vi "5790A acdc unit.vi"(6 "error in":errorcluster, 8 "unit":enum16{"ppm", "pct", "V", "ratio"}(ring), 9 "5790A":refnum<visa-resource-name>) -> (0 "error out":errorcluster, 3 "Session Out":refnum<visa-resource-name>)   [LabVIEW 2009]
uses:
  <vilib>/Instr/_visa.llb/VISA GPIB Control REN Mode.ctl
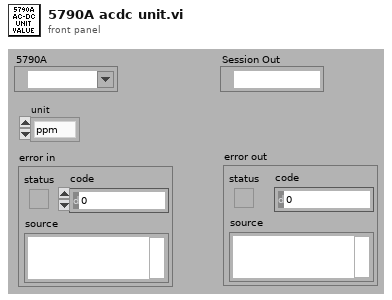
[diagram p1: front panel]
types:
  T1 = typedef "VISA GPIB Control REN Mode.ctl" = u16
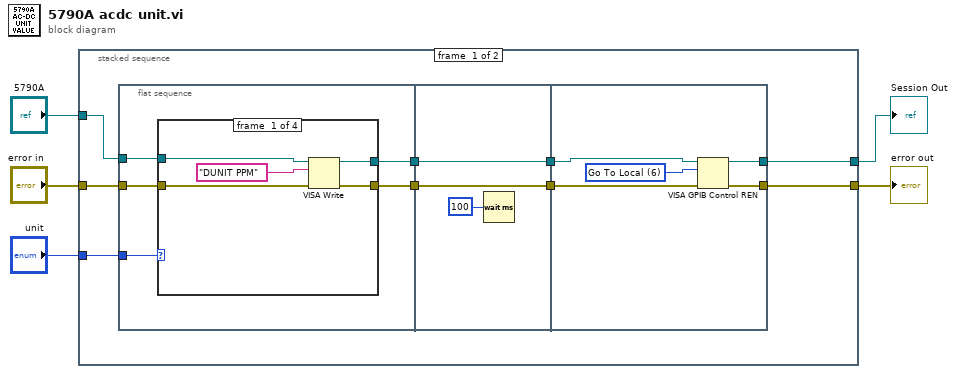
[diagram p0: block diagram]
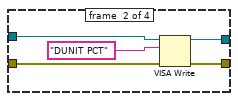
[diagram p2: hidden frame]
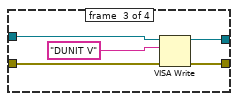
[diagram p3: hidden frame]
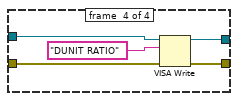
[diagram p4: hidden frame]
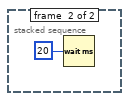
[diagram p5: hidden frame]
diagram:
  n1 = stacked-sequence {
    tunnel: "5790A" -> [w14 _]
    tunnel: "error in" -> [w13 _]
    tunnel: [w12 _] -> w4
    tunnel: [w11 _] -> w5
    tunnel: "unit" -> [w10 _]
    frame #0 {
      n2 = flat-sequence {
        tunnel: w10 -> [w19]
        tunnel: w13 -> [w17]
        tunnel: w14 -> [w18]
        tunnel: [w16] -> w8
        tunnel: [w15] -> w6
        tunnel: [w41] -> w9
        tunnel: w8 -> [w41]
        tunnel: [w40] -> w7
        tunnel: w6 -> [w40]
        tunnel: [w46] -> w11
        tunnel: [w45] -> w12
        tunnel: w9 -> [w44]
        tunnel: w7 -> [w43]
        frame #0 {
          n3 = case shown="\"pct\"" w19 {
            tunnel: w18 -> [w21 w28 w33 w36]
            tunnel: w17 -> [w22 w27 w32 w35]
            tunnel: [w24 w25 w30 w38] -> w16
            tunnel: [w23 w26 w31 w37] -> w15
            frame #0 {
              n4 = VISA Write(VISA resource name=w21, write buffer="DUNIT PPM", error in (no error)=w22) -> (VISA resource name out=w24:refnum<visa-resource-name>, error out=w23:errorcluster)  [unwired: 1 out]
            }
            frame #1 {
              n5 = VISA Write(VISA resource name=w28, write buffer="DUNIT PCT", error in (no error)=w27) -> (VISA resource name out=w25:refnum<visa-resource-name>, error out=w26:errorcluster)  [unwired: 1 out]
            }
            frame #2 {
              n6 = VISA Write(VISA resource name=w33, write buffer="DUNIT V", error in (no error)=w32) -> (VISA resource name out=w30:refnum<visa-resource-name>, error out=w31:errorcluster)  [unwired: 1 out]
            }
            frame #3 {
              n7 = VISA Write(VISA resource name=w36, write buffer="DUNIT RATIO", error in (no error)=w35) -> (VISA resource name out=w38:refnum<visa-resource-name>, error out=w37:errorcluster)  [unwired: 1 out]
            }
          }
        }
        frame #1 {
          n8 = Wait (ms)(milliseconds to wait=u32 100 ("millisecond multiple")) -> ()  [unwired: 1 out]
        }
        frame #2 {
          w47 = T1 6 items=["Deassert REN", "Assert REN", "Go To Local; Deassert REN ", "Assert REN; Address Device", "Local Lockout (Addressed Devices)", "Local Lockout (This Device)", "Go To Local"] ("Mode")
          n9 = VISA GPIB Control REN(8:w43, 10:w47, 11:w44) -> (0:w45:errorcluster, 3:w46:refnum<visa-resource-name>)
        }
      }
    }
    frame #1 {
      n10 = Wait (ms)(milliseconds to wait=u32 20 ("millisecond multiple")) -> ()  [unwired: 1 out]
    }
  }
  "Session Out" <- w5
  "error out" <- w4
